vi "measurements.vi"() -> ()   [LabVIEW 2024]
uses:
  AGH/Dydaktyka/Przedmioty/Moje/MiSP/Wyposazenie/Soft/WaveRecorder/UserInterfaceTypedefs.llb/MainDataStruct.ctl
  AGH/Dydaktyka/Przedmioty/Moje/MiSP/Wyposazenie/Soft/WaveRecorder/UserInterfaceTypedefs.llb/MeasurementResult.ctl
  AGH/Dydaktyka/Przedmioty/Moje/MiSP/Wyposazenie/Soft/WaveRecorder/MeasurementTypedefs.llb/ChannelMsmResults.ctl
  AGH/Dydaktyka/Przedmioty/Moje/MiSP/Wyposazenie/Soft/WaveRecorder/RedrawUI_Typedefs.llb/ResponseAnnotationArray.ctl
  AGH/Dydaktyka/Przedmioty/Moje/MiSP/Wyposazenie/Soft/WaveRecorder/RedrawUI_Typedefs.llb/ResponseAnnotation.ctl
  AGH/Dydaktyka/Przedmioty/Moje/MiSP/Wyposazenie/Soft/WaveRecorder/FormulasTypedefs.llb/VirtualChannels.ctl
  AGH/Dydaktyka/Przedmioty/Moje/MiSP/Wyposazenie/Soft/WaveRecorder/FormulasTypedefs.llb/Constants.ctl
  AGH/Dydaktyka/Przedmioty/Moje/MiSP/Wyposazenie/Soft/WaveRecorder/FormulasTypedefs.llb/Formulas.ctl
  AGH/Dydaktyka/Przedmioty/Moje/MiSP/Wyposazenie/Soft/WaveRecorder/UserInterfaceTypedefs.llb/ValidArea.ctl
  AGH/Dydaktyka/Przedmioty/Moje/MiSP/Wyposazenie/Soft/WaveRecorder/MeasurementTypedefs.llb/MeasurementSettingsV1.ctl
  AGH/Dydaktyka/Przedmioty/Moje/MiSP/Wyposazenie/Soft/WaveRecorder/UserInterfaceTypedefs.llb/ChannellParams.ctl
  AGH/Dydaktyka/Przedmioty/Moje/MiSP/Wyposazenie/Soft/WaveRecorder/MeasurementTypedefs.llb/AcquisitionParams.ctl
  <vilib>/Utility/file.llb/Write Delimited Spreadsheet (DBL).vi
panel:
  in  "DataStructure":T1={"Current measur."=-1, "MsmInProgress ?"=FALSE, "Measurements"=[], "Display mode"=enum."Compare Channel", "Current channel"=0, "ConstantsCurrentRow"=0, "FormulasCurrentRow"=0, "ShowAnnotations?"=FALSE, "VirtualChannels"={"Parameters"={"names"=[]}, "Formulas"=[]}, "Selection"={"Begin"=0.0, "End"=10.0}, "MeasurementSettings"={"ChannellsParams"=[], "Name"="", "AcquisitionsParams"={"Frequency"=0.0, "Time"=0.0, "Scope"=enum."+/-10"}, "Description"=""}}
  # "Voltage"
  # "[V]"
  # "Acquisition"
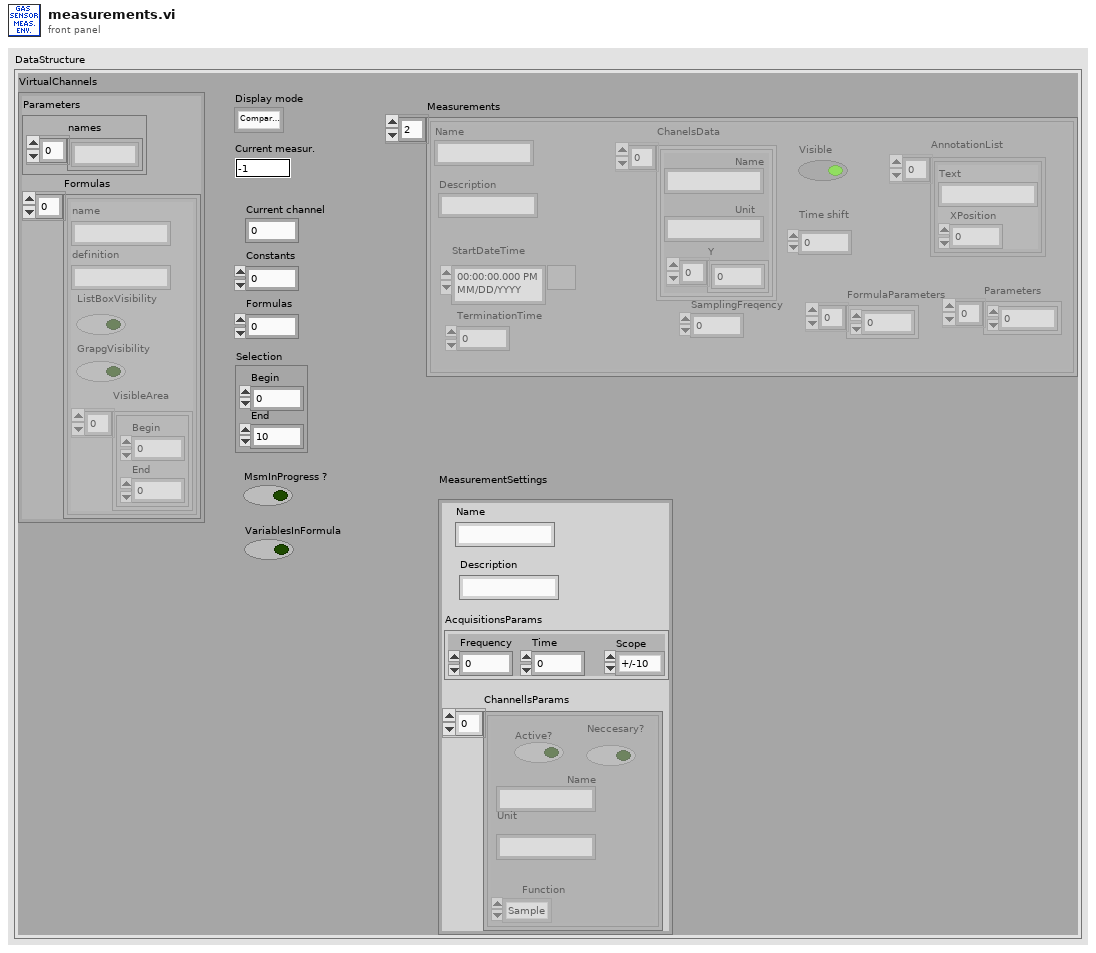
[diagram p1: front panel]
types:
  T1 = typedef "MainDataStruct.ctl" = cluster{"Current measur.":i32, "MsmInProgress ?":bool, "Measurements":T2[], "Display mode":enum32{"Compare Measur.", "Compare Channel", "Single Chart"}, "Current channel":u8, "ConstantsCurrentRow":u8, "FormulasCurrentRow":u8, "ShowAnnotations?":bool, "VirtualChannels":T6, "Selection":cluster{"Begin":sgl, "End":sgl}, "MeasurementSettings":T10}
  T2 = typedef "MeasurementResult.ctl" = cluster{"Name":string, "Visible":bool, "Time shift":dbl, "ChanelsData":T3[], "StartDateTime":timestamp, "AnnotationList":T4, "Description":string, "FormulaParameters":dbl[], "TerminationTime":u32, "Parameters":dbl[], "SamplingFreqency":u32}
  T3 = typedef "ChannelMsmResults.ctl" = cluster{"Y":dbl[], "Name":string, "Unit":string}
  T4 = typedef "ResponseAnnotationArray.ctl" = T5[]
  T5 = typedef "ResponseAnnotation.ctl" = cluster{"Text":string, "XPosition":dbl}
  T6 = typedef "VirtualChannels.ctl" = cluster{"Parameters":T7, "Formulas":T8[]}
  T7 = typedef "Constants.ctl" = cluster{"names":string[]}
  T8 = typedef "Formulas.ctl" = cluster{"name":string, "definition":string, "ListBoxVisibility":bool, "GrapgVisibility":bool, "VisibleArea":T9[]}
  T9 = typedef "ValidArea.ctl" = cluster{"Begin":sgl, "End":sgl}
  T10 = typedef "MeasurementSettingsV1.ctl" = cluster{"ChannellsParams":T11[], "Name":string, "AcquisitionsParams":T12, "Description":string}
  T11 = typedef "ChannellParams.ctl" = cluster{"Name":string, "Function":enum16{"Light", "Sample", "Si", "SiHg"}, "Active?":bool, "Unit":string, "Neccesary?":bool}
  T12 = typedef "AcquisitionParams.ctl" = cluster{"Frequency":dbl, "Time":dbl, "Scope":enum16{"+/-0,2", "+/-1", "+/-5", "+/-10"}}
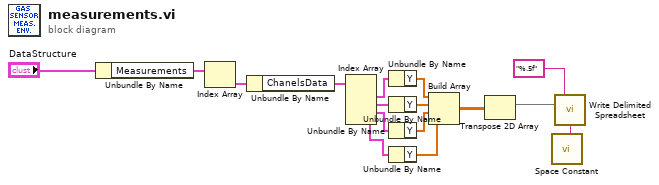
[diagram p0: block diagram]
diagram:
  n1 = Unbundle By Name("DataStructure") -> ("Measurements"=w15:T2[])
  n2 = Index Array(array=w15) -> (element=w14:T2)  [unwired: 1 in]
  n3 = Unbundle By Name(w14) -> ("ChanelsData"=w13:T3[])
  n4 = Index Array(array=w13) -> (element #1=w12:T3, element #2=w11:T3, element #3=w10:T3, element #4=w2:T3)  [unwired: 4 in]
  n5 = Unbundle By Name(w12) -> ("Y"=w9:dbl[])
  n6 = Unbundle By Name(w11) -> ("Y"=w8:dbl[])
  n7 = Unbundle By Name(w10) -> ("Y"=w7:dbl[])
  n8 = Unbundle By Name(w2) -> ("Y"=w1:dbl[])
  n9 = Build Array(w9, w8, w7, w1) -> (w6:dbl[][])
  n10 = Transpose 2D Array(2D array=w6) -> (transposed array=w5:dbl[][])
  n11 = call <vilib>:"Space Constant.vi"() -> ("String"=w4:string)
  n12 = call-poly <vilib>:"Write Delimited Spreadsheet.vi"("format (%.3f)"="%.5f", "2D data"=w5, "delimiter (\\t)"=w4) -> ()  [unwired: 11 in, 2 out]
